vi "Day 14-2.vi"() -> ()   [LabVIEW 2020]
panel:
  out "x-y 2":dbl
  out "x-y":i64
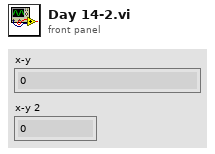
[diagram p1: front panel]
types:
  T1 = typedef "Puzzle 14-2.ctl" = cluster{"Sequence":u8[], "Histogram":i64[], "Poly Map":u8[], "Pairs":i64[]}
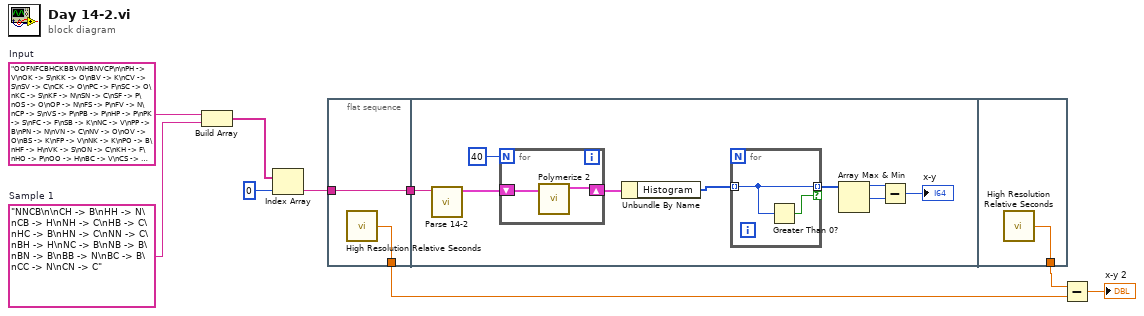
[diagram p0: block diagram]
diagram:
  w8 = "NNCB\n\nCH -> B\nHH -> N\nCB -> H\nNH -> C\nHB -> C\nHC -> B\nHN -> C\nNN -> C\nBH -> H\nNC -> B\nNB -> B\nBN -> B\nBB -> N\nBC -> B\nCC -> N\nCN -> C"  # Sample 1
  w9 = "OOFNFCBHCKBBVNHBNVCP\n\nPH -> V\nOK -> S\nKK -> O\nBV -> K\nCV -> S\nSV -> C\nCK -> O\nPC -> F\nSC -> O\nKC -> S\nKF -> N\nSN -> C\nSF -> P\nOS -> O\nOP -> N\nFS -> P\nFV -> N\nCP -> S\nVS -> P\nPB -> P\nHP -> P\nPK -> S\nFC -> F\nSB -> K\nNC -> V\nPP -> B\nPN -> N\nVN -> C\nNV -> O\nOV -> O\nBS -> K\nFP -> V\nNK -> K\nPO -> B\nHF -> H\nVK -> S\nON -> C\nKH -> F\nHO -> P\nOO -> H\nBC -> V\nCS -> O\nOC -> B\nVB -> N\nOF -> P\nFK -> H\nOH -> H\nCF -> K\nCC -> V\nBK -> O\nBH -> F\nVV -> N\nKS -> V\nFO -> F\nSH -> F\nOB -> O\nVH -> F\nHH -> P\nPF -> C\nNF -> V\nVP -> S\nCN -> V\nSK -> O\nFB -> S\nFN -> S\nBF -> H\nFF -> V\nCB -> P\nNN -> O\nVC -> F\nHK -> F\nBO -> H\nKO -> C\nCH -> N\nKP -> C\nHS -> P\nNP -> O\nNS -> V\nNB -> H\nHN -> O\nBP -> C\nVF -> S\nKN -> P\nHC -> C\nPS -> K\nBB -> O\nNO -> N\nNH -> F\nBN -> F\nKV -> V\nSS -> K\nCO -> H\nKB -> P\nFH -> C\nSP -> C\nSO -> V\nPV -> S\nVO -> O\nHV -> N\nHB -> V"  # Input
  n1 = Build Array(w9, w8) -> (w7:string[])
  n2 = Index Array(array=w7, index=0) -> (element=w5:string)
  n3 = flat-sequence {
    tunnel: w5 -> [w11]
    tunnel: [w11] -> w4
    tunnel: [w10] -> w2
    tunnel: w4 -> [w20]
    tunnel: [w25] -> w3
    frame #0 {
      n4 = call <vilib>:"High Resolution Relative Seconds.vi"() -> ("relative seconds"=w10:dbl)
    }
    frame #1 {
      n5 = call "Parse 14-2.vi"("String"=w20) -> ("Puzzle"=w19:T1)  [unwired: 10 in]
      n6 = for {
        N: 40 -> [_]
        shift-right: [w21] -> w17
        shift-left: w19 -> [w22]
        n7 = call "Polymerize 2.vi"("Puzzle In"=w22) -> ("Puzzle"=w21:T1)  [unwired: 10 in]
      }
      n8 = Unbundle By Name(w17) -> ("Histogram"=w13:i64[])
      n9 = for {
        tunnel: w13 -> [w24] mode=indexing
        tunnel: [w24] -> w12 mode=indexing if=w23
        n10 = Greater Than 0?(x=w24) -> (x > 0?=w23:bool)
      }
      n11 = Array Max & Min(array=w12) -> (max value=w16:i64, min value=w15:i64)  [unwired: 2 out]
      n12 = Subtract(x=w16, y=w15) -> (x-y=→"x-y":i64)
    }
    frame #2 {
      n13 = call <vilib>:"High Resolution Relative Seconds.vi"() -> ("relative seconds"=w25:dbl)
    }
  }
  n14 = Subtract(x=w3, y=w2) -> (x-y=→"x-y 2":dbl)
